vi "TRANS_To_Data.vi"(10 "Size":T2, 11 "String":string) -> (3 "Bin Data":T1)   [LabVIEW 2017]
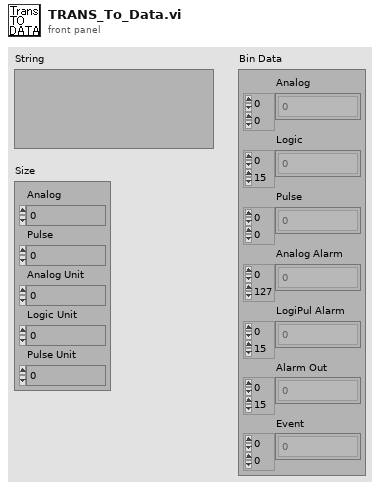
[diagram p1: front panel]
types:
  T1 = cluster{"Analog":i16[][], "Logic":u8[][], "Pulse":i32[][], "Analog Alarm":u8[][], "LogiPul Alarm":u8[][], "Alarm Out":u8[][], "Event":u8[][]}
  T2 = cluster{"Analog":i32, "Pulse":i32, "Analog Unit":i32, "Logic Unit":i32, "Pulse Unit":i32}
  T3 = cluster{i16[][], "Bit[]":u8[][], i32[][], "Bit[]":u8[][], "Bit[]":u8[][], "Bit[]":u8[][], "Bit[]":u8[][]}
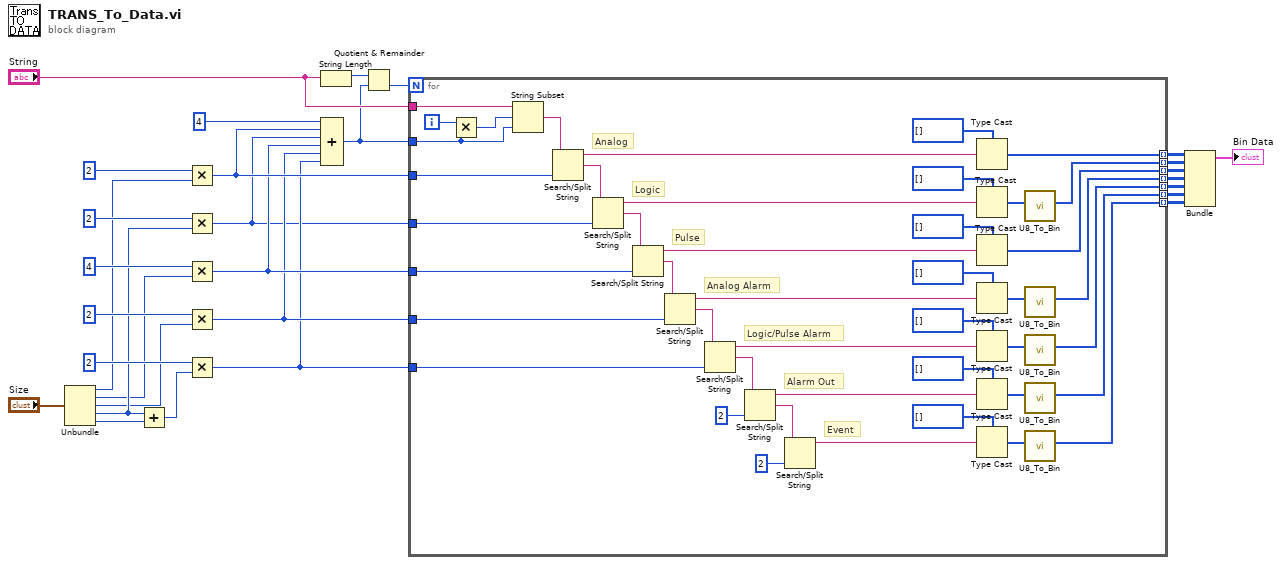
[diagram p0: block diagram]
diagram:
  n1 = Unbundle("Size") -> ("Analog"=w14:i32, "Pulse"=w3:i32, "Analog Unit"=w2:i32, "Logic Unit"=w4:i32, "Pulse Unit"=w1:i32)
  n2 = Add(x=w4, y=w1) -> (x+y=w13:i32)
  n3 = Multiply(x=2 ("y"), y=w14) -> (x*y=w27:i32)
  n4 = Multiply(x=2 ("y"), y=w4) -> (x*y=w16:i32)
  n5 = Multiply(x=4 ("y"), y=w3) -> (x*y=w26:i32)
  n6 = Multiply(x=2 ("y"), y=w2) -> (x*y=w20:i32)
  n7 = Multiply(x=2 ("y"), y=w13) -> (x*y=w19:i32)
  n8 = String Length(string="String") -> (length=w24:i32)
  n9 = Compound Arithmetic op=ADD(4 ("value"), w27, w16, w26, w20, w19) -> (w21:i32)
  n10 = Quotient & Remainder(x=w24, y=w21) -> (floor(x/y)=w23:i32)  [unwired: 1 out]
  n11 = for {
    N: w23 -> [_]
    tunnel: w27 -> [w47]
    tunnel: w16 -> [w46]
    tunnel: w26 -> [w45]
    tunnel: w20 -> [w44]
    tunnel: w19 -> [w43]
    tunnel: "String" -> [w39]
    tunnel: w21 -> [w41]
    tunnel: [w31] -> w12 mode=indexing
    tunnel: [w37] -> w11 mode=indexing
    tunnel: [w36] -> w10 mode=indexing
    tunnel: [w35] -> w9 mode=indexing
    tunnel: [w34] -> w8 mode=indexing
    tunnel: [w33] -> w7 mode=indexing
    tunnel: [w32] -> w6 mode=indexing
    i -> [w40]
    # "Event"
    # "Alarm Out"
    # "Logic/Pulse Alarm"
    # "Analog Alarm"
    # "Pulse"
    # "Logic"
    # "Analog"
    n12 = Multiply(x=w40, y=w41) -> (x*y=w42:i32)
    n13 = String Subset(string=w39, offset (0)=w42, length (rest)=w41) -> (substring=w38:string)
    n14 = Search/Split String(string=w38, offset (0)=w47) -> (substring before match=w74:string, match + rest of string=w73:string)  [unwired: 1 in, 1 out]
    n15 = Search/Split String(string=w73, offset (0)=w46) -> (substring before match=w72:string, match + rest of string=w71:string)  [unwired: 1 in, 1 out]
    n16 = Search/Split String(string=w71, offset (0)=w45) -> (substring before match=w70:string, match + rest of string=w69:string)  [unwired: 1 in, 1 out]
    n17 = Search/Split String(string=w69, offset (0)=w44) -> (substring before match=w68:string, match + rest of string=w65:string)  [unwired: 1 in, 1 out]
    n18 = Search/Split String(string=w65, offset (0)=w43) -> (substring before match=w67:string, match + rest of string=w64:string)  [unwired: 1 in, 1 out]
    n19 = Search/Split String(string=w64, offset (0)=2) -> (substring before match=w66:string, match + rest of string=w62:string)  [unwired: 1 in, 1 out]
    n20 = Search/Split String(string=w62, offset (0)=2) -> (substring before match=w61:string)  [unwired: 1 in, 2 out]
    n21 = Type Cast(type=i16[] [], x=w74) -> (*(type *) &x=w31:i16[])
    n22 = Type Cast(type=u16[] [], x=w72) -> (*(type *) &x=w48:u16[])
    n23 = Type Cast(type=i32[] [], x=w70) -> (*(type *) &x=w36:i32[])
    n24 = Type Cast(type=u16[] [], x=w68) -> (*(type *) &x=w50:u16[])
    n25 = Type Cast(type=u16[] [], x=w67) -> (*(type *) &x=w49:u16[])
    n26 = Type Cast(type=u16[] [], x=w66) -> (*(type *) &x=w52:u16[])
    n27 = Type Cast(type=u16[] [], x=w61) -> (*(type *) &x=w51:u16[])
    n28 = call "U8_To_Bin.vi"("U16[]"=w48) -> ("Bit[]"=w37:u8[])  [unwired: 10 out]
    n29 = call "U8_To_Bin.vi"("U16[]"=w50) -> ("Bit[]"=w35:u8[])  [unwired: 10 out]
    n30 = call "U8_To_Bin.vi"("U16[]"=w49) -> ("Bit[]"=w34:u8[])  [unwired: 10 out]
    n31 = call "U8_To_Bin.vi"("U16[]"=w52) -> ("Bit[]"=w33:u8[])  [unwired: 10 out]
    n32 = call "U8_To_Bin.vi"("U16[]"=w51) -> ("Bit[]"=w32:u8[])  [unwired: 10 out]
  }
  n33 = Bundle(w12, "Bit[]"=w11, w10, "Bit[]"=w9, "Bit[]"=w8, "Bit[]"=w7, "Bit[]"=w6) -> (→"Bin Data":T3)  [unwired: 1 out]
